vi "Scroll Bar State.vi"(8 "error in (no error)":errorcluster, 9 "Vertical Scrollbar Visibility":T1(ring)=enum."Off While Running", 11 "reference":refnum<vi>) -> (0 "error out":errorcluster)   [LabVIEW 2018]
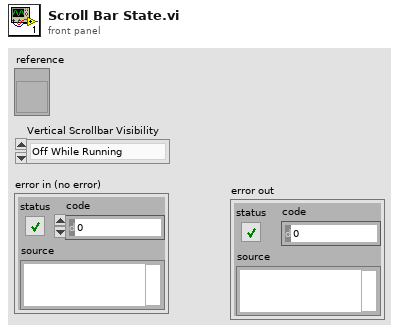
[diagram p1: front panel]
types:
  T1 = enum16{"Always On", "Always Off", "Off While Running"}
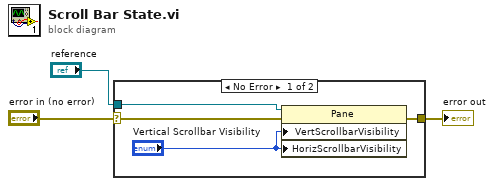
[diagram p0: block diagram]
diagram:
  n1 = case shown="No Error" "error in (no error)" {
    selector: "error in (no error)" -> [w6 w8]
    tunnel: [w5 w8] -> w2
    tunnel: "reference" -> [w4 _]
    frame No Error {
      n2 = property on="Property Node" class="Pane"(reference=w4, error in=w6, "VertScrollbarVisibility"="Vertical Scrollbar Visibility", "HorizScrollbarVisibility"="Vertical Scrollbar Visibility") -> (error out=w5:errorcluster)  [unwired: 1 out]
    }
    frame Error {
    }
  }
  "error out" <- w2
